vi "Ex 1.vi"() -> ()   [LabVIEW 2021]
panel:
  out "deg F":dbl
  in  "deg C":dbl
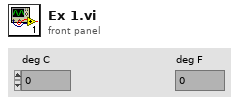
[diagram p1: front panel]
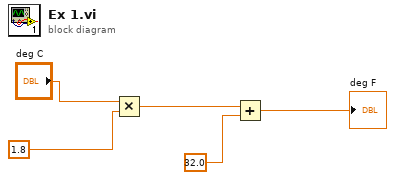
[diagram p0: block diagram]
diagram:
  n1 = Multiply(x="deg C", y=1.8 ("x*y")) -> (x*y=w2:dbl)
  n2 = Add(x=w2, y=32.0) -> (x+y=→"deg F":dbl)
